vi "Pickup HDI.vi"(8 "error in":errorcluster, 10 "Slot Number":u32, 11 "PickupTool in":refnum<class "PickupTool Class.lvclass">) -> (0 "error out":errorcluster, 3 "PickupTool out":refnum<class "PickupTool Class.lvclass">)   [LabVIEW 2011, in "PickupTool Class.lvclass"]
uses:
  PickupTool Class.lvclass
  WorkTable Class/WorkTable Class.lvclass
  Vec3d Class/Vec3d Class.lvclass
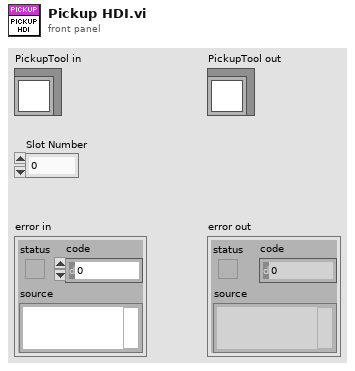
[diagram p1: front panel]
types:
  T1 = typedef "Worktable_HDI Slot.ctl" = cluster{"HDI Assembly State":enum16{"Empty", "Populated"}, "HDI Type":enum16{"HDI", "Polyimide"}, "Vacuum Channel":u32, "Location/Orientation":T2}
  T2 = typedef "Position_Orientation.ctl" = cluster{"Center":refnum<class "Vec3d Class.lvclass">, "Orientation":refnum<class "Orient3d Class.lvclass">}
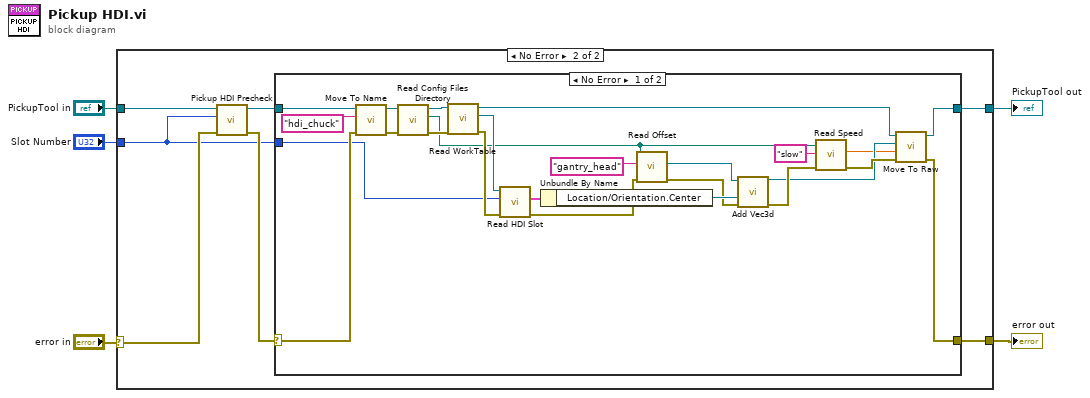
[diagram p0: block diagram]
diagram:
  n1 = case shown="No Error" "error in" {
    selector: "error in" -> [w6 w13]
    tunnel: [w6 w12] -> w4
    tunnel: [w7 w11] -> w2
    tunnel: "PickupTool in" -> [w7 w14]
    tunnel: "Slot Number" -> [_ w8]
    frame Error {
    }
    frame No Error {
      n2 = call "Pickup HDI Precheck.vi"("error in"=w13, "Slot Number in"=w8, "PickupTool Class in"=w14) -> ("error out"=w9:errorcluster, "PickupTool Class out"=w10:refnum<class "PickupTool Class.lvclass">)  [unwired: 7 in]
      n3 = case shown="No Error" w9 {
        selector: w9 -> [w37 w41]
        tunnel: [w26 w41] -> w12
        tunnel: w10 -> [w39 w40]
        tunnel: [w27 w40] -> w11
        tunnel: w8 -> [w34 _]
        frame No Error {
          n4 = call-dynamic "Move To Name.vi"("error in"=w37, "Destination Name"="hdi_chuck", "Gantry in"=w39) -> ("error out"=w23:errorcluster, "Gantry out"=w24:refnum<class "PickupTool Class.lvclass">)  [unwired: 7 in]
          n5 = call-dynamic "Read Config Files Directory.vi"("error in (no error)"=w23, "Gantry Class in"=w24) -> ("error out"=w22:errorcluster, "Config Files Directory"=w15:path, "Gantry Class out"=w25:refnum<class "PickupTool Class.lvclass">)  [unwired: 7 in]
          n6 = call-dynamic "Read WorkTable.vi"("error in"=w22, "Gantry Class in"=w25) -> ("error out"=w35:errorcluster, "WorkTable Class.lvclass"=w36:refnum<class "WorkTable Class.lvclass">, "Gantry Class out"=w16:refnum<class "PickupTool Class.lvclass">)  [unwired: 7 in]
          n7 = call-dynamic "Read HDI Slot.vi"("error in"=w35, "HDI Slot Number"=w34, "WorkTable in"=w36) -> ("error out"=w19:errorcluster, "HDI Slot"=w33:T1)  [unwired: 6 in, 1 out]
          n8 = Unbundle By Name(w33) -> ("Location/Orientation.Center"=w30:refnum<class "Vec3d Class.lvclass">)
          n9 = call "Read Offset.vi"("error in"=w19, "Offset Name"="gantry_head", "Config Folder"=w15) -> ("error out"=w18:errorcluster, "Vec3d out"=w20:refnum<class "Vec3d Class.lvclass">)  [unwired: 7 in]
          n10 = call-dynamic "Add Vec3d.vi"("error in (no error)"=w18, 10:"Vec3d Class in"=w30, 11:"Vec3d Class in"=w20) -> ("error out"=w29:errorcluster, "Vec3d Class out"=w28:refnum<class "Vec3d Class.lvclass">)  [unwired: 7 in]
          n11 = call "Read Speed.vi"("error in"=w29, "Speeds Label"="slow", "Config Files Path"=w15) -> ("error out"=w32:errorcluster, "Speed"=w17:dbl)  [unwired: 7 in]
          n12 = call-dynamic "Move To Raw.vi"("error in"=w32, "Speed"=w17, "Destination"=w28, "Gantry in"=w16) -> ("error out"=w26:errorcluster, "Gantry out"=w27:refnum<class "PickupTool Class.lvclass">)  [unwired: 6 in]
        }
        frame Error {
        }
      }
    }
  }
  "error out" <- w4
  "PickupTool out" <- w2
